vi "MT EbN0 Calculation(FSK).vi"(0 "Recieved waveform":T3={"t0"=0.0, "dt"=1.0, "Y"=[]} {"Y" format="%.3f"; "dt" format="%^.2e"; "t0" format="%.4f"}, 1 "pulse shaping filter coefficients":dbl[](array[numeric]) format="%.2f", 5 "FSK system parameters":T2={"samples per symbol (16)"=16, "symbol map"=[], "symbol phase continuity"=enum."continuous"} {"symbol map" format="%.2f"}, 7 "synchronization parameters":T1 {"sync sequence" format="%.2f"}, 9 "matched filter coefficients":dbl[](array[numeric]) format="%.2f", 11 "error in (no error)":errorcluster, 12 "reset? (T)":bool=TRUE) -> (4 "Eb/N0":dbl, 6 "Eb/N0(dB)":dbl, 15 "error out":errorcluster)   [LabVIEW 2020, in "niDMT.lvlib"]
uses:
  <vilib>/addons/Modulation/niDMT.lvlib
  <vilib>/addons/Modulation/Analog/controls/Complex Data Waveform.ctl
  <vilib>/addons/Modulation/niAMT.lvlib
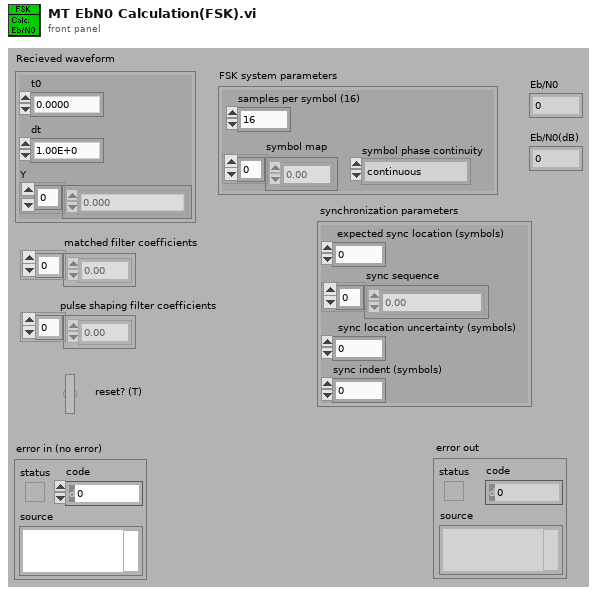
[diagram p1: front panel]
types:
  T1 = cluster{"expected sync location (symbols)":i32, "sync sequence":cdb[], "sync location uncertainty (symbols)":i32, "sync indent (symbols)":i32}
  T2 = cluster{"samples per symbol (16)":i32, "symbol map":dbl[], "symbol phase continuity":enum16{"continuous", "discontinuous"}}
  T3 = typedef "niAMT.lvlib/Complex Data Waveform.ctl" = cluster{"t0":dbl, "dt":dbl, "Y":cdb[]}
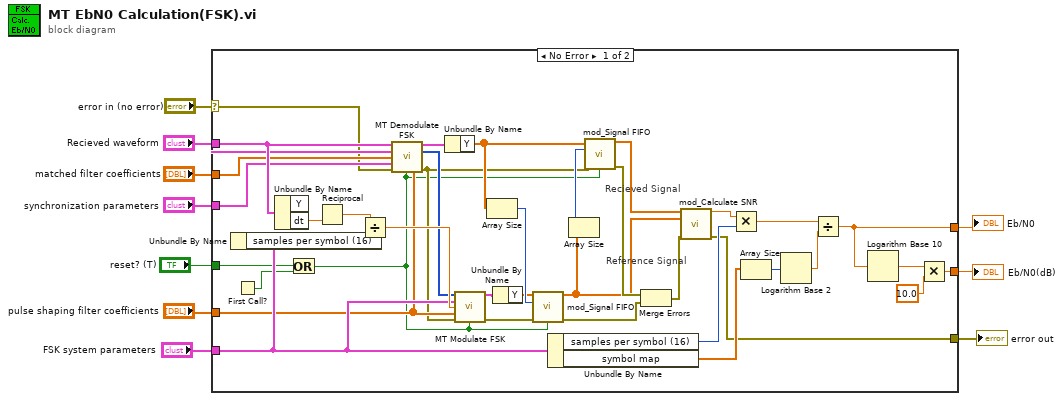
[diagram p0: block diagram]
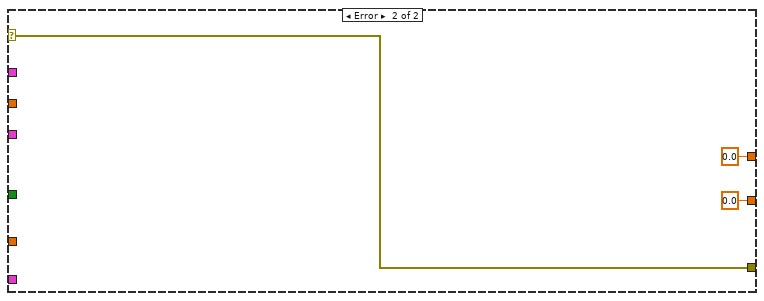
[diagram p2: hidden frame]
diagram:
  n1 = case shown="No Error" "error in (no error)" {
    selector: "error in (no error)" -> [w14 w49]
    tunnel: "Recieved waveform" -> [w41 _]
    tunnel: "FSK system parameters" -> [w40 _]
    tunnel: "synchronization parameters" -> [w39 _]
    tunnel: "matched filter coefficients" -> [w38 _]
    tunnel: "pulse shaping filter coefficients" -> [w37 _]
    tunnel: [w27 0.0] -> w5
    tunnel: [w24 0.0] -> w4
    tunnel: [w16 w49] -> w3
    tunnel: "reset? (T)" -> [w13 _]
    frame No Error {
      # "Recieved Signal"
      # "Reference Signal"
      n2 = Unbundle By Name(w40) -> ("samples per symbol (16)"=w46:i32)
      n3 = First Call?() -> (First Call?: T/F=w12:bool)
      n4 = Unbundle By Name(w41) -> ("dt"=w48:dbl)  [unwired: 1 out]
      n5 = Or(x=w13, y=w12) -> (x .or. y?=w11:bool)
      n6 = Reciprocal(x=w48) -> (1/x=w44:dbl)
      n7 = Divide(x=w44, y=w46) -> (x/y=w47:dbl)
      n8 = call <vilib>:"MT Demodulate FSK.vi"("input complex waveform"=w41, "FSK system parameters"=w40, "matched filter coefficients"=w38, "synchronization parameters"=w39, "error in (no error)"=w14, "pulse shaping filter coefficients"=w37, "reset? (T)"=w11) -> ("recovered complex waveform"=w34:T3, "output bit stream"=w36:i8[], "error out"=w23:errorcluster)  [unwired: 6 out]
      n9 = Unbundle By Name(w34) -> ("Y"=w32:cdb[])
      n10 = call <vilib>:"MT Modulate FSK.vi"("input bit stream"=w36, "FSK system parameters"=w40, "symbol rate (Hz)"=w47, "pulse shaping filter coefficients"=w37, "error in (no error)"=w23, "reset? (T)"=w11) -> ("output complex waveform"=w33:T3, "error out"=w22:errorcluster)  [unwired: 1 in, 7 out]
      n11 = Array Size(array=w32) -> (size(s)=w31:i32)
      n12 = Unbundle By Name(w33) -> ("Y"=w30:cdb[])
      n13 = call <vilib>:"mod_Signal FIFO.vi"("Signal In"=w30, "Output Length"=w31, "error in (no error)"=w22, "Reset? (T)"=w11) -> ("Signal Out"=w18:cdb[], "error out"=w20:errorcluster)  [unwired: 10 out]
      n14 = Unbundle By Name(w40) -> ("samples per symbol (16)"=w45:i32, "symbol map"=w43:dbl[])
      n15 = Array Size(array=w18) -> (size(s)=w29:i32)
      n16 = call <vilib>:"mod_Signal FIFO.vi"("Signal In"=w32, "Output Length"=w29, "error in (no error)"=w23, "Reset? (T)"=w11) -> ("Signal Out"=w19:cdb[], "error out"=w21:errorcluster)  [unwired: 10 out]
      n17 = Merge Errors(w21, w20) -> (w17:errorcluster)
      n18 = call <vilib>:"mod_Calculate SNR.vi"("Recieved Waveform"=w19, "Reference Waveform"=w18, "error in (no error)"=w17) -> ("SNR"=w15:dbl, "error out"=w16:errorcluster)  [unwired: 11 out]
      n19 = Multiply(x=w15, y=w45) -> (x*y=w35:dbl)
      n20 = Array Size(array=w43) -> (size(s)=w42:i32)
      n21 = Logarithm Base 2(1:w42) -> (0:w28:dbl)
      n22 = Divide(x=w35, y=w28) -> (x/y=w27:dbl)
      n23 = Logarithm Base 10(1:w27) -> (0:w26:dbl)
      n24 = Multiply(x=w26, y=10.0) -> (x*y=w24:dbl)
    }
    frame Error {
    }
  }
  "Eb/N0" <- w5
  "Eb/N0(dB)" <- w4
  "error out" <- w3
